vi "3.1.11-Calibration Function.vi"() -> ()   [LabVIEW 2010]
uses:
  2-Low Neurons/2.1-Act Command Typedef.ctl
  2-Low Neurons/2.1 PID Gains Typedef.ctl
  2-Low Neurons/2.1 Act Debug.ctl
  <vilib>/rvi/interface/nirviReadWriteControl/nirviReadWriteControl.xnode
  2-Low Neurons/2-FPGA VI Typedef.ctl
  FPGA Bitfiles/DaveBrain_FPGATarget_1-Hindbrain_F0E489D8.lvbitx
  1-Hindbrain.vi
  <vilib>/rvi/interface/common/niFpgaNodeNameForErrorReporting.ctl
  <vilib>/rvi/errors/niLvFpgaWhatHappensToTopLevelVI.ctl
  3.0-Global.vi
  <vilib>/RVI Host/nirviSupport.llb/nirviErrorClusterFromErrorCode.vi
  <vilib>/rvi/errors/niLvFpgaAdjustHostInterfaceError.vi
panel:
  in  "Steering Move Rate":i32
  in  "User want to get on with his life":bool
  out "Lidar Position Integer @ Home":i32
  out "Lidar Motor Position Integer @ Home":i32
  out "Positive Inflexion Point":bool
  out "Waveform Chart":dbl[](graph)
  out "2.1 Act Debug":T1
  out "2.1 Act Command":T2={"Inhibit All Motors"=FALSE, "2.1 Direct Override"=FALSE, "Drive Speed Integer Setpoint"=0, "Steering Integer Setpoint"=0, "Lidar Position Integer Setpoint"=0, "Drive Direct"=0.0, "Steer Direct"=0.0, "Lidar Direct "=0.0, "2.1.3 Drive PID Gains"={"P Gain"=0.25, "I Gain"=0.25, "D Gain"=0.25, "P Gain - Exp"=2, "I Gain - Exp"=2, "D Gain - Exp"=2, "I Saturate"=0.25}, "Drive Limit"=0.0, "2.1.2 Steering Input C"=0.0, "2.1.2 Steering Input K"=0.0} {"2.1.2 Steering Input K" format="%_10e"; "2.1.2 Steering Input C" format="%_10e"; "2.1.3 Drive PID Gains"."I Saturate" format="%#_14g"; "2.1.3 Drive PID Gains"."P Gain" format="%.8f"; "2.1.3 Drive PID Gains"."I Gain" format="%.8f"; "2.1.3 Drive PID Gains"."D Gain" format="%.8f"}
  in  "Stop":bool
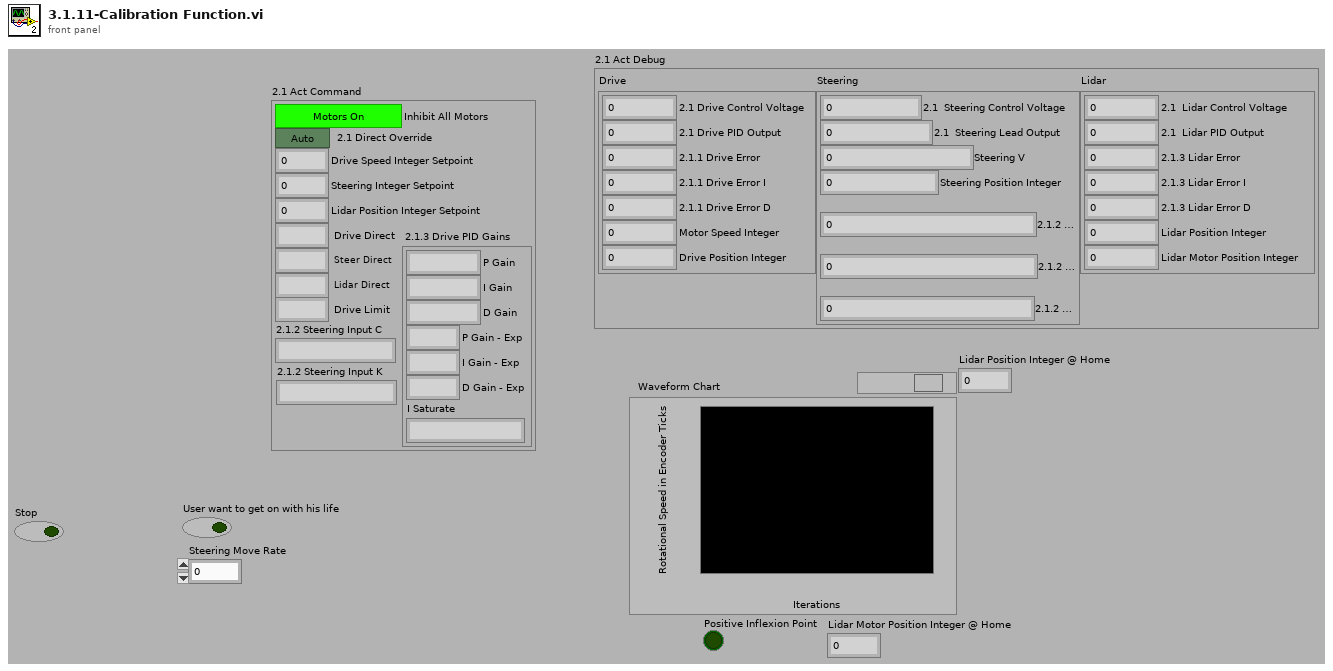
[diagram p1: front panel]
types:
  T1 = typedef "2.1 Act Debug.ctl" = cluster{"Drive":cluster{"2.1 Drive Control Voltage":fxp<+/-,20,5>, "2.1 Drive PID Output":fxp<+/-,20,5>, "2.1.1 Drive Error":fxp<+/-,18,1>, "2.1.1 Drive Error I":fxp<+/-,64,46>, "2.1.1 Drive Error D":fxp<+/-,18,1>, "Motor Speed Integer":fxp<+/-,10,8>, "Drive Position Integer":i32}, "Steering":cluster{"2.1  Steering Control Voltage":fxp<+/-,20,5>, "2.1  Steering Lead Output":fxp<+/-,20,5>, "Steering V":fxp<+/-,10,8>, "Steering Position Integer":i32, "2.1.2 sqrt(10)s+bdt":fxp<+/-,18,20>, "2.1.2 (sqrt(10)s+bdt)/(s/sqrt(10)+bdt)":fxp<+/-,20,22>, "2.1.2 s(sqrt(10)s+bdt)/(s/sqrt(10)+bdt)":fxp<+/-,20,22>}, "Lidar":cluster{"2.1  Lidar Control Voltage":fxp<+/-,20,5>, "2.1  Lidar PID Output":fxp<+/-,20,5>, "2.1.3 Lidar Error":fxp<+/-,18,1>, "2.1.3 Lidar Error I":fxp<+/-,64,46>, "2.1.3 Lidar Error D":fxp<+/-,18,1>, "Lidar Position Integer":i32, "Lidar Motor Position Integer":i32}}
  T2 = typedef "2.1-Act Command Typedef.ctl" = cluster{"Inhibit All Motors":bool, "2.1 Direct Override":bool, "Drive Speed Integer Setpoint":i32, "Steering Integer Setpoint":i32, "Lidar Position Integer Setpoint":i32, "Drive Direct":fxp<+/-,20,5>, "Steer Direct":fxp<+/-,20,5>, "Lidar Direct ":fxp<+/-,20,5>, "2.1.3 Drive PID Gains":T3, "Drive Limit":fxp<+/-,20,5>, "2.1.2 Steering Input C":fxp<+,8,-2>, "2.1.2 Steering Input K":fxp<+/-,14,-6>}
  T3 = typedef "2.1 PID Gains Typedef.ctl" = cluster{"P Gain":fxp<+/-,18,1>, "I Gain":fxp<+/-,18,1>, "D Gain":fxp<+/-,18,1>, "P Gain - Exp":i8, "I Gain - Exp":i8, "D Gain - Exp":i8, "I Saturate":fxp<+/-,64,46>}
  T4 = enum16{"Set Lidar Rotation", "Wait for Lidar Crossover Point", "Stop Lidar, Set Global", "Set Tentative Steering Zero", "Move Setpoint Left", "Move Setpoint Right", "Re-Calibrate Steering Zero"}
  T5 = typedef "niFpgaNodeNameForErrorReporting.ctl" = enum16{"Open FPGA VI Reference", "Read/Write Control", "Invoke Method: Abort", "Invoke Method: Acknowledge IRQ", "Invoke Method: Download", "Invoke Method: FIFO.Configure", "Invoke Method: FIFO.Read", "Invoke Method: FIFO.Start", "Invoke Method: FIFO.Stop", "Invoke Method: FIFO.Write", "Invoke Method: Reset", "Invoke Method: Run", "Invoke Method: Wait on IRQ", "Close FPGA VI Reference"}
  T6 = typedef "niLvFpgaWhatHappensToTopLevelVI.ctl" = enum16{"top level VI scripted behind XNode", "top level VI inlined behind XNode"}
  T7 = typedef "2-FPGA VI Typedef.ctl" = refnum<k20>
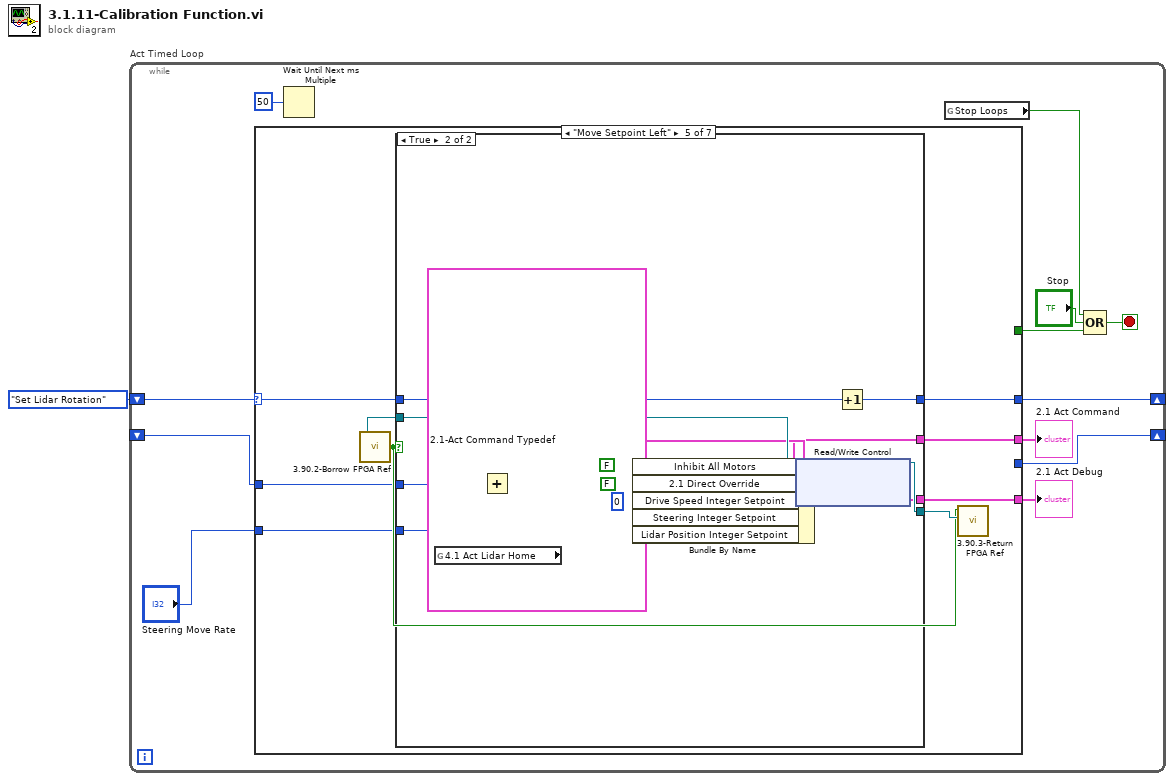
[diagram p0: block diagram]
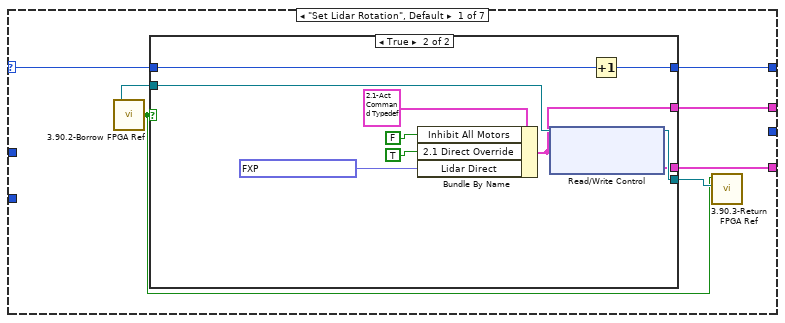
[diagram p2: hidden frame]
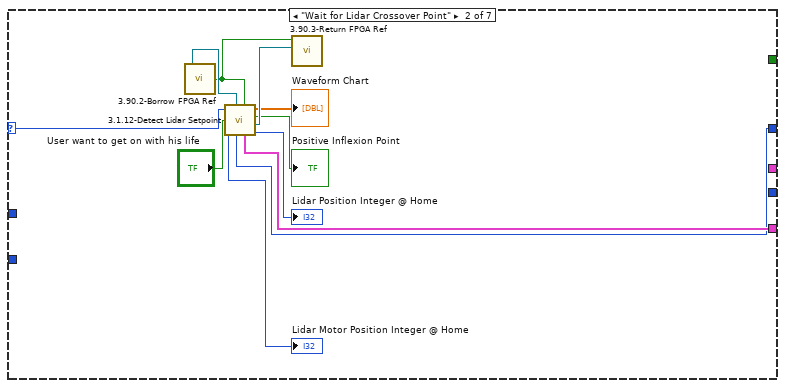
[diagram p4: hidden frame]
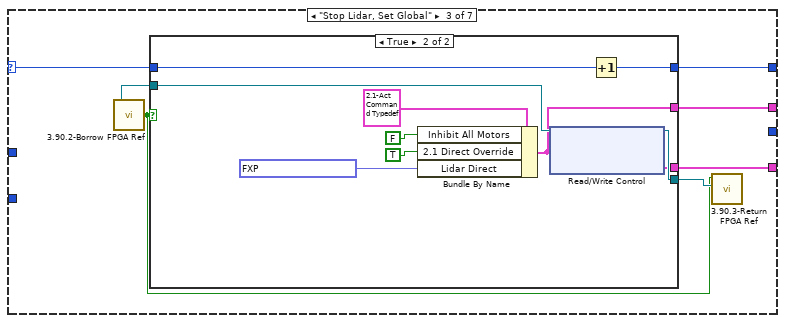
[diagram p5: hidden frame]
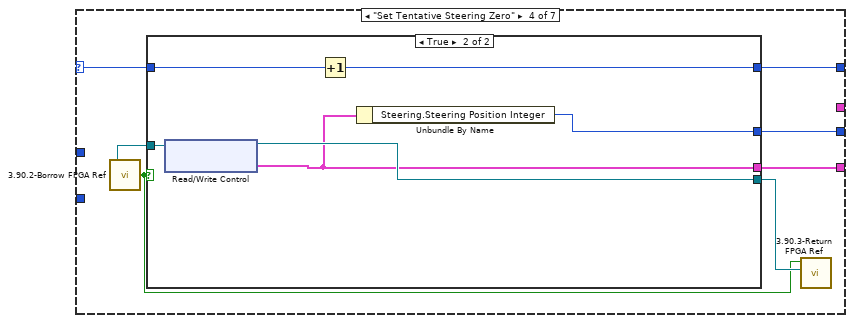
[diagram p7: hidden frame]
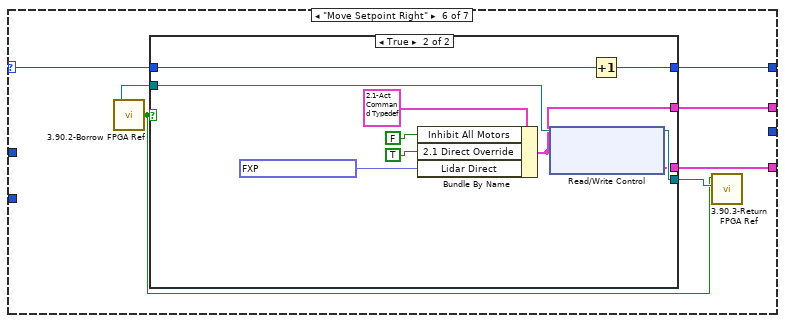
[diagram p10: hidden frame]
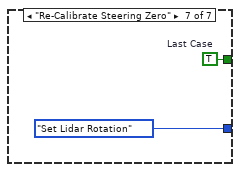
[diagram p12: hidden frame]
diagram:
  n1 = while "Act Timed Loop" {
    shift-right: [w5] -> _
    shift-left: T4."Set Lidar Rotation" -> [w8]
    shift-right: [w4] -> _
    shift-left: _ -> [w3]
    stop <- w12 stop-if-true
    n2 = case shown="\"Move Setpoint Left\"" w8 {
      selector: w8 -> [w15 w65 w71 w117 w154 w203 _]
      tunnel: [_ _ _ _ _ _ w248] -> w9
      tunnel: [w17 _ w73 _ w156 w205 _] -> w7
      tunnel: [w16 w66 w72 w118 w155 w204 _] -> w6
      tunnel: [w14 w64 w70 w116 w153 w202 T4."Set Lidar Rotation"] -> w5
      tunnel: [_ _ _ w115 _ _ _] -> w4
      tunnel: w3 -> [_ _ _ _ w152 _ _]
      tunnel: "Steering Move Rate" -> [_ _ _ _ w151 _ _]
      frame "Set Lidar Rotation", Default {
        n3 = call "3.90.2-Borrow FPGA Ref.vi"() -> ("Has Refrence"=w18:bool, "Ref Out"=w19:T7)
        n4 = case shown="True" w18 {
          tunnel: w19 -> [w22 w32]
          tunnel: [w22 w31] -> w20
          tunnel: [_ w26] -> w17
          tunnel: [_ w25] -> w16
          tunnel: w15 -> [w21 w24]
          tunnel: [w21 w23] -> w14
          frame False {
          }
          frame True {
            n5 = Bundle By Name(cluster=T2 {"Inhibit All Motors"=FALSE, "2.1 Direct Override"=FALSE, "Drive Speed Integer Setpoint"=0, "Steering Integer Setpoint"=0, "Lidar Position Integer Setpoint"=0, "Drive Direct"=0.0, "Steer Direct"=0.0, "Lidar Direct "=0.0, "2.1.3 Drive PID Gains"={"P Gain"=0.0, "I Gain"=0.0, "D Gain"=0.0, "P Gain - Exp"=0, "I Gain - Exp"=0, "D Gain - Exp"=0, "I Saturate"=0.0}, "Drive Limit"=0.0, "2.1.2 Steering Input C"=0.0, "2.1.2 Steering Input K"=0.0} ("2.1 Act Command"), "Inhibit All Motors"=FALSE, "2.1 Direct Override"=TRUE, "Lidar Direct"=fxp<+/-,20,5> 1.0) -> (w26:T2)
            n6 = xnode "Read/Write Control"("FPGA VI Reference In"=w32, "2.1 Act Command"=w26) -> ("FPGA VI Reference Out"=w31:T7, "2.1 Act Debug"=w25:T1)  [unwired: 1 in, 1 out]
            n7 = Increment(x=w24) -> (x+1=w23:T4)
          }
        }
        n8 = call "3.90.3-Return FPGA Ref.vi"("element"=w20, "Has Refrence"=w18) -> ()  [unwired: 3 in]
      }
      frame "Wait for Lidar Crossover Point" {
        n9 = call "3.90.2-Borrow FPGA Ref.vi"() -> ("Has Refrence"=w67:bool, "Ref Out"=w68:T7)
        n10 = call "3.1.12-Detect Lidar Setpoint.vi"("Enum 2"=w65, "Ref Out"=w68, "User want to get on with his life"="User want to get on with his life", "Has Refrence"=w67) -> ("Lidar Motor Position Integer @ Home"=→"Lidar Motor Position Integer @ Home":i32, "Enum"=w64:T4, "Waveform Chart"=→"Waveform Chart":dbl[], "Positive Inflexion Point"=→"Positive Inflexion Point":bool, "2.1 Act Debug"=w66:T1, "FPGA VI Reference Out"=w69:T7, "Lidar Position Integer @ Home"=→"Lidar Position Integer @ Home":i32)
        n11 = call "3.90.3-Return FPGA Ref.vi"("element"=w69, "Has Refrence"=w67) -> ()  [unwired: 3 in]
      }
      frame "Stop Lidar, Set Global" {
        n12 = call "3.90.2-Borrow FPGA Ref.vi"() -> ("Has Refrence"=w74:bool, "Ref Out"=w75:T7)
        n13 = case shown="True" w74 {
          tunnel: w75 -> [w78 w88]
          tunnel: [w78 w87] -> w76
          tunnel: [_ w82] -> w73
          tunnel: [_ w81] -> w72
          tunnel: w71 -> [w77 w80]
          tunnel: [w77 w79] -> w70
          frame False {
          }
          frame True {
            n14 = Bundle By Name(cluster=T2 {"Inhibit All Motors"=FALSE, "2.1 Direct Override"=FALSE, "Drive Speed Integer Setpoint"=0, "Steering Integer Setpoint"=0, "Lidar Position Integer Setpoint"=0, "Drive Direct"=0.0, "Steer Direct"=0.0, "Lidar Direct "=0.0, "2.1.3 Drive PID Gains"={"P Gain"=0.0, "I Gain"=0.0, "D Gain"=0.0, "P Gain - Exp"=0, "I Gain - Exp"=0, "D Gain - Exp"=0, "I Saturate"=0.0}, "Drive Limit"=0.0, "2.1.2 Steering Input C"=0.0, "2.1.2 Steering Input K"=0.0} ("2.1 Act Command"), "Inhibit All Motors"=FALSE, "2.1 Direct Override"=TRUE, "Lidar Direct"=fxp<+/-,20,5> 0.0) -> (w82:T2)
            n15 = xnode "Read/Write Control"("FPGA VI Reference In"=w88, "2.1 Act Command"=w82) -> ("FPGA VI Reference Out"=w87:T7, "2.1 Act Debug"=w81:T1)  [unwired: 1 in, 1 out]
            n16 = Increment(x=w80) -> (x+1=w79:T4)
          }
        }
        n17 = call "3.90.3-Return FPGA Ref.vi"("element"=w76, "Has Refrence"=w74) -> ()  [unwired: 3 in]
      }
      frame "Set Tentative Steering Zero" {
        n18 = call "3.90.2-Borrow FPGA Ref.vi"() -> ("Has Refrence"=w119:bool, "Ref Out"=w120:T7)
        n19 = case shown="True" w119 {
          tunnel: w120 -> [w123 w126]
          tunnel: [w123 w129] -> w121
          tunnel: [_ w125] -> w118
          tunnel: w117 -> [w122 w128]
          tunnel: [w122 w127] -> w116
          tunnel: [_ w124] -> w115
          frame False {
          }
          frame True {
            n20 = xnode "Read/Write Control"("FPGA VI Reference In"=w126) -> ("FPGA VI Reference Out"=w129:T7, "2.1 Act Debug"=w125:T1)  [unwired: 1 in, 1 out]
            n21 = Increment(x=w128) -> (x+1=w127:T4)
            n22 = Unbundle By Name(w125) -> ("Steering.Steering Position Integer"=w124:i32)
          }
        }
        n23 = call "3.90.3-Return FPGA Ref.vi"("element"=w121, "Has Refrence"=w119) -> ()  [unwired: 3 in]
      }
      frame "Move Setpoint Left" {
        n24 = call "3.90.2-Borrow FPGA Ref.vi"() -> ("Has Refrence"=w157:bool, "Ref Out"=w158:T7)
        n25 = case shown="True" w157 {
          tunnel: w158 -> [w161 w175]
          tunnel: [w161 w174] -> w159
          tunnel: [_ w170] -> w156
          tunnel: [_ w169] -> w155
          tunnel: w154 -> [w160 w168]
          tunnel: [w160 w167] -> w153
          tunnel: w152 -> [_ w164]
          tunnel: w151 -> [_ w162]
          frame False {
          }
          frame True {
            n26 = global read "3.0-Global.vi" "4.1 Act Lidar Home"() -> (w166:i32)
            n27 = Add(x=w162, y=w164) -> (x+y=w163:i32)
            n28 = Bundle By Name(cluster=T2 {"Inhibit All Motors"=FALSE, "2.1 Direct Override"=FALSE, "Drive Speed Integer Setpoint"=0, "Steering Integer Setpoint"=0, "Lidar Position Integer Setpoint"=0, "Drive Direct"=0.0, "Steer Direct"=0.0, "Lidar Direct "=0.0, "2.1.3 Drive PID Gains"={"P Gain"=0.0, "I Gain"=0.0, "D Gain"=0.0, "P Gain - Exp"=0, "I Gain - Exp"=0, "D Gain - Exp"=0, "I Saturate"=0.0}, "Drive Limit"=0.0, "2.1.2 Steering Input C"=0.0, "2.1.2 Steering Input K"=0.0} ("2.1 Act Command"), "Inhibit All Motors"=FALSE, "2.1 Direct Override"=FALSE, "Drive Speed Integer Setpoint"=0, "Steering Integer Setpoint"=w163, "Lidar Position Integer Setpoint"=w166) -> (w170:T2)
            n29 = xnode "Read/Write Control"("FPGA VI Reference In"=w175, "2.1 Act Command"=w170) -> ("FPGA VI Reference Out"=w174:T7, "2.1 Act Debug"=w169:T1)  [unwired: 1 in, 1 out]
            n30 = Increment(x=w168) -> (x+1=w167:T4)
          }
        }
        n31 = call "3.90.3-Return FPGA Ref.vi"("element"=w159, "Has Refrence"=w157) -> ()  [unwired: 3 in]
      }
      frame "Move Setpoint Right" {
        n32 = call "3.90.2-Borrow FPGA Ref.vi"() -> ("Has Refrence"=w206:bool, "Ref Out"=w207:T7)
        n33 = case shown="True" w206 {
          tunnel: w207 -> [w210 w220]
          tunnel: [w210 w219] -> w208
          tunnel: [_ w214] -> w205
          tunnel: [_ w213] -> w204
          tunnel: w203 -> [w209 w212]
          tunnel: [w209 w211] -> w202
          frame False {
          }
          frame True {
            n34 = Bundle By Name(cluster=T2 {"Inhibit All Motors"=FALSE, "2.1 Direct Override"=FALSE, "Drive Speed Integer Setpoint"=0, "Steering Integer Setpoint"=0, "Lidar Position Integer Setpoint"=0, "Drive Direct"=0.0, "Steer Direct"=0.0, "Lidar Direct "=0.0, "2.1.3 Drive PID Gains"={"P Gain"=0.0, "I Gain"=0.0, "D Gain"=0.0, "P Gain - Exp"=0, "I Gain - Exp"=0, "D Gain - Exp"=0, "I Saturate"=0.0}, "Drive Limit"=0.0, "2.1.2 Steering Input C"=0.0, "2.1.2 Steering Input K"=0.0} ("2.1 Act Command"), "Inhibit All Motors"=FALSE, "2.1 Direct Override"=TRUE, "Lidar Direct"=fxp<+/-,20,5> 1.0) -> (w214:T2)
            n35 = xnode "Read/Write Control"("FPGA VI Reference In"=w220, "2.1 Act Command"=w214) -> ("FPGA VI Reference Out"=w219:T7, "2.1 Act Debug"=w213:T1)  [unwired: 1 in, 1 out]
            n36 = Increment(x=w212) -> (x+1=w211:T4)
          }
        }
        n37 = call "3.90.3-Return FPGA Ref.vi"("element"=w208, "Has Refrence"=w206) -> ()  [unwired: 3 in]
      }
      frame "Re-Calibrate Steering Zero" {
        w248 = TRUE  # Last Case
      }
    }
    "2.1 Act Command" <- w7
    "2.1 Act Debug" <- w6
    n38 = Wait Until Next ms Multiple(millisecond multiple=u32 50) -> ()  [unwired: 1 out]
    n39 = global read "3.0-Global.vi" "Stop Loops"() -> (w10:bool)
    n40 = Compound Arithmetic op=OR(w10, "Stop", w9) -> (w12:bool)
  }
